vi "findCamerasInUse.vi"(8 "error in (no error)":errorcluster, 11 "ScriptListCompiler in":refnum<class "ScriptListCompiler.lvclass">) -> (0 "error out":errorcluster, 2 "camerasInScript":enum16{"Pixis", "ProEM", "PixelFly"}[](array[ring]), 3 "ScriptListCompiler out":refnum<class "ScriptListCompiler.lvclass">)   [LabVIEW 2011, in "Compiler.lvlib" / "ScriptListCompiler.lvclass"]
uses:
  ScriptListCompiler.lvclass
  ScriptListCompiler.lvclass/ScriptListCompiler.ctl
  Scripting/ScriptingEvent/ScriptEventList/ScriptEventList.lvclass
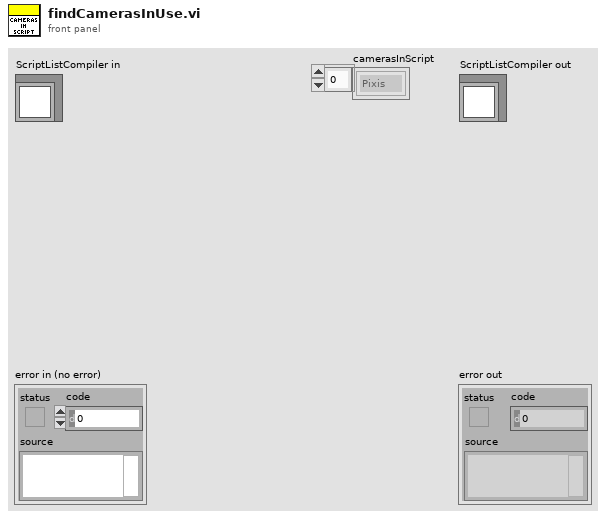
[diagram p1: front panel]
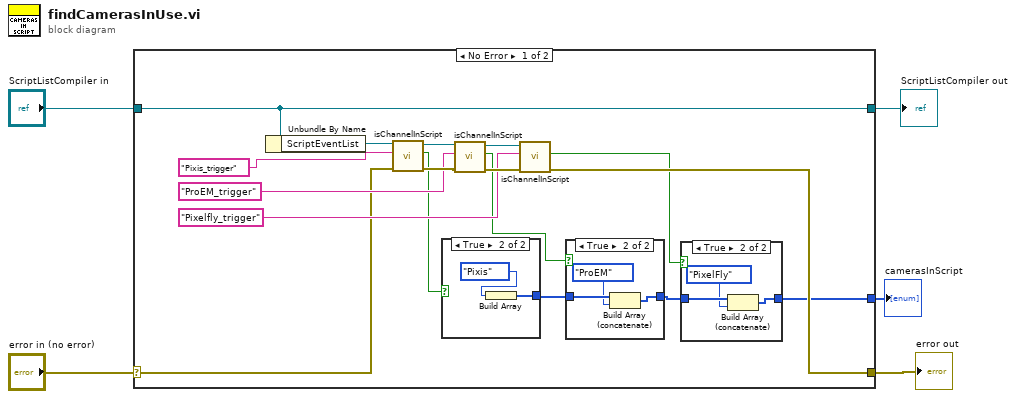
[diagram p0: block diagram]
diagram:
  n1 = case shown="No Error" "error in (no error)" {
    selector: "error in (no error)" -> [w13 w34]
    tunnel: [w12 w34] -> w4
    tunnel: [w22 w33] -> w2
    tunnel: "ScriptListCompiler in" -> [w22 w33]
    tunnel: [w6 _] -> w1
    frame No Error {
      n2 = Unbundle By Name(w22) -> ("ScriptEventList"=w21:refnum<class "ScriptEventList.lvclass">)
      n3 = call "isChannelInScript.vi"("error in (no error)"=w13, "channelName"="Pixis_trigger", "ScriptEventList in"=w21) -> ("error out"=w18:errorcluster, "found Channel"=w11:bool, "ScriptEventList out"=w20:refnum<class "ScriptEventList.lvclass">)  [unwired: 6 in]
      n4 = case shown="True" w11 {
        tunnel: [_ w31] -> w10
        frame False {
        }
        frame True {
          n5 = Build Array(enum16{"Pixis", "ProEM", "PixelFly"}."Pixis" ("Camera")) -> (w31:enum16{"Pixis", "ProEM", "PixelFly"}[])
        }
      }
      n6 = call "isChannelInScript.vi"("error in (no error)"=w18, "channelName"="ProEM_trigger", "ScriptEventList in"=w20) -> ("error out"=w17:errorcluster, "found Channel"=w9:bool, "ScriptEventList out"=w19:refnum<class "ScriptEventList.lvclass">)  [unwired: 6 in]
      n7 = call "isChannelInScript.vi"("error in (no error)"=w17, "channelName"="Pixelfly_trigger", "ScriptEventList in"=w19) -> ("error out"=w12:errorcluster, "found Channel"=w8:bool)  [unwired: 6 in, 1 out]
      n8 = case shown="True" w9 {
        tunnel: [w27 w30] -> w7
        tunnel: w10 -> [w27 w29]
        frame False {
        }
        frame True {
          n9 = Build Array (concatenate)(w29, enum16{"Pixis", "ProEM", "PixelFly"}."ProEM" ("Camera")) -> (w30:enum16{"Pixis", "ProEM", "PixelFly"}[])
        }
      }
      n10 = case shown="True" w8 {
        tunnel: [w23 w26] -> w6
        tunnel: w7 -> [w23 w25]
        frame False {
        }
        frame True {
          n11 = Build Array (concatenate)(w25, enum16{"Pixis", "ProEM", "PixelFly"}."PixelFly" ("Camera")) -> (w26:enum16{"Pixis", "ProEM", "PixelFly"}[])
        }
      }
    }
    frame Error {
    }
  }
  "error out" <- w4
  "ScriptListCompiler out" <- w2
  "camerasInScript" <- w1
